vi "SDO_TRAJECTORY_GET_CLOSED_LOOP.vi"() -> (3 "AUTO_CLOSED_LOOP":bool)   [LabVIEW 2019]
uses:
  PPS_TRAJECTORY_GLOBALS.vi
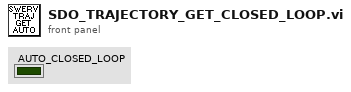
[diagram p1: front panel]
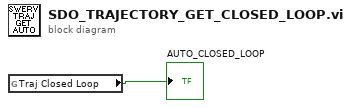
[diagram p0: block diagram]
diagram:
  n1 = global read "PPS_TRAJECTORY_GLOBALS.vi" "Traj Closed Loop"() -> (→"AUTO_CLOSED_LOOP":bool)
